vi "Validate Receive SubAddress.vi"(6 "RT 1?":bool, 8 "error in (no error)":errorcluster, 11 "RT Config in":refnum<class "RT Config.lvclass">) -> (0 "error out":errorcluster, 3 "RT Config out":refnum<class "RT Config.lvclass">)   [LabVIEW 2016, in "RT Config.lvclass"]
uses:
  RT Config.lvclass
  PPLs/FPGA Interface.lvlibp/FPGA Interface/FPGA Interface.lvclass
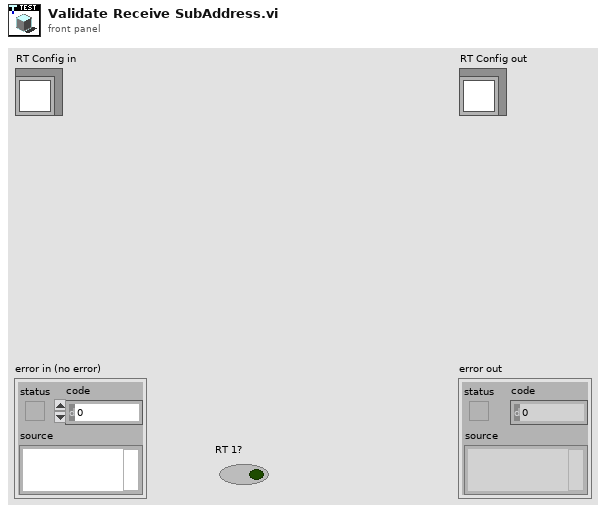
[diagram p1: front panel]
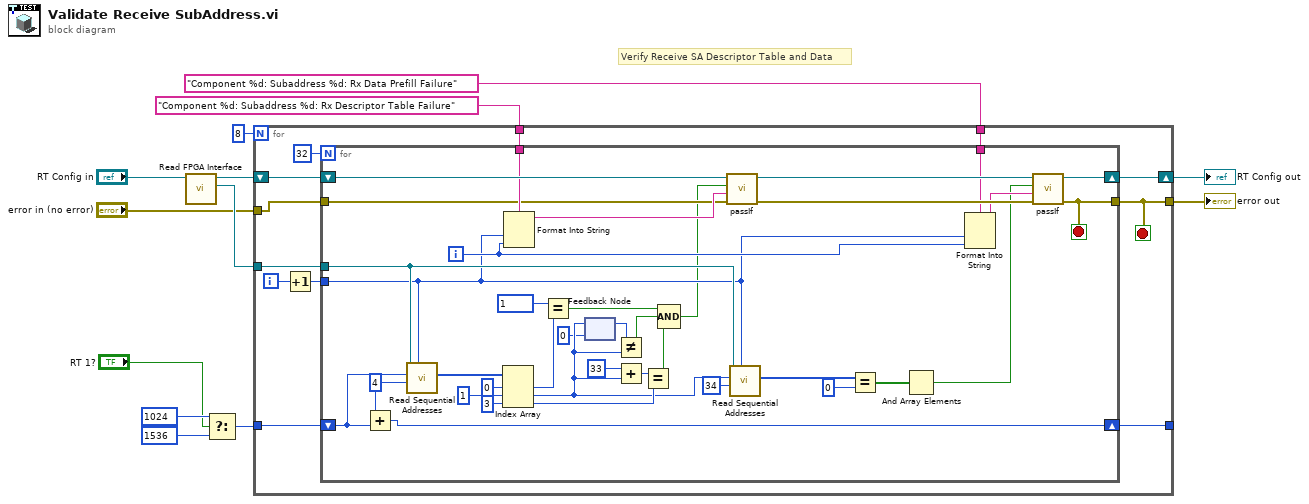
[diagram p0: block diagram]
diagram:
  # "Verify Receive SA Descriptor Table and Data"
  n1 = call-dynamic "Read FPGA Interface.vi"("1553 Test in"="RT Config in") -> ("FPGA Interface"=w13:refnum<class "FPGA Interface.lvclass">, "1553 Test out"=w9:refnum<class "RT Config.lvclass">)  [unwired: 8 in, 1 out]
  n2 = Select(t=u16 1024, s="RT 1?", f=u16 1536) -> (s? t:f=w10:u16)
  n3 = for {
    N: 8 -> [_]
    tunnel: w13 -> [w22]
    shift-right: [w19] -> w3
    shift-left: w9 -> [w20]
    tunnel: "Component %d: Subaddress %d: Rx Descriptor Table Failure" ("message (\"\")") -> [w18]
    tunnel: w10 -> [w24]
    tunnel: [w23] -> _
    tunnel: [w16] -> w2
    tunnel: "error in (no error)" -> [w15]
    tunnel: "Component %d: Subaddress %d: Rx Data Prefill Failure" ("message (\"\")") -> [w14]
    i -> [w25]
    stop <- w16 stop-if-true
    n4 = Increment(x=w25) -> (x+1=w21:i32)
    n5 = for {
      N: 32 -> [_]
      tunnel: w22 -> [w55]
      tunnel: w21 -> [w43]
      tunnel: w18 -> [w53]
      shift-right: [w60] -> w23
      shift-left: w24 -> [w61]
      shift-right: [w49] -> w19
      shift-left: w20 -> [w54]
      tunnel: [w47] -> w16
      tunnel: w15 -> [w46]
      tunnel: w14 -> [w45]
      i -> [w44]
      stop <- w47 stop-if-true
      w62 = u16 4 ("Addresses to Read")
      n6 = Add(x=w62, y=w61) -> (x+y=w60:u16)
      n7 = call-dynamic "Read Sequential Addresses.vi"("Target IC (1-8)"=w43, "Addresses to Read"=w62, "Starting Address"=w61, "FPGA Interface in"=w55) -> ("Data"=w59:u16[])  [unwired: 6 in, 1 out]
      n8 = Index Array(array=w59, index #1=0 ("index"), index #2=1 ("index"), index #3=3 ("index")) -> (element #1=w36:u16, element #2=w31:u16, element #3=w32:u16)
      n9 = Format Into String(format string=w53, w43, w44) -> (resulting string=w52:string)  [unwired: 2 in, 1 out]
      n10 = Equal?(x=u16 1, y=w36) -> (x = y?=w39:bool)
      n11 = feedback-in #1(w31) -> ()
      n12 = feedback #1(u16 0 ("Data")) -> (w38:u16)
      n13 = Not Equal?(x=w38, y=w31) -> (x != y?=w37:bool)
      n14 = Add(x=u16 33, y=w31) -> (x+y=w34:u16)
      n15 = Equal?(x=w34, y=w32) -> (x = y?=w33:bool)
      n16 = Compound Arithmetic op=AND(w39, w37, w33) -> (w40:bool)
      n17 = call-dynamic "passIf.vi"("error in (no error)"=w46, "message (\"\")"=w52, "pass"=w40, "TestCase in"=w54) -> ("error out"=w48:errorcluster, "TestCase out"=w50:refnum<class "RT Config.lvclass">)  [unwired: 6 in]
      n18 = call-dynamic "Read Sequential Addresses.vi"("Target IC (1-8)"=w43, "Addresses to Read"=u16 34, "Starting Address"=w31, "FPGA Interface in"=w55) -> ("Data"=w30:u16[])  [unwired: 6 in, 1 out]
      n19 = Equal?(x=w30, y=u16 0 ("Data")) -> (x = y?=w28:bool[])
      n20 = And Array Elements(Boolean array=w28) -> (logical AND=w27:bool)
      n21 = Format Into String(format string=w45, w43, w44) -> (resulting string=w42:string)  [unwired: 2 in, 1 out]
      n22 = call-dynamic "passIf.vi"("error in (no error)"=w48, "message (\"\")"=w42, "pass"=w27, "TestCase in"=w50) -> ("error out"=w47:errorcluster, "TestCase out"=w49:refnum<class "RT Config.lvclass">)  [unwired: 6 in]
    }
  }
  "error out" <- w2
  "RT Config out" <- w3
